vi "getColorMode.vi"(9 "wColorPatternDESC":u16, 10 "wRoiX0":u16, 11 "wRoiY0":u16) -> (3 "colorMode":i32)   [LabVIEW 2020]
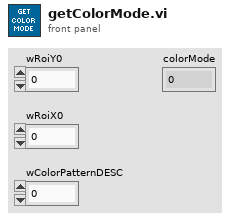
[diagram p1: front panel]
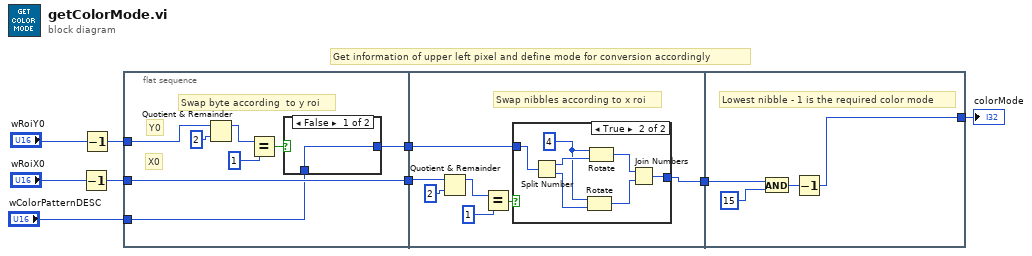
[diagram p0: block diagram]
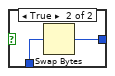
[diagram p2: hidden frame]
diagram:
  # "Get information of upper left pixel and define mode for conversion accordingly"
  n1 = Decrement(x="wRoiX0") -> (x-1=w4:u16)
  n2 = Decrement(x="wRoiY0") -> (x-1=w2:u16)
  n3 = flat-sequence {
    tunnel: w4 -> [w15]
    tunnel: w2 -> [w17]
    tunnel: [w15] -> w9
    tunnel: [w11] -> w8
    tunnel: "wColorPatternDESC" -> [w10]
    tunnel: w9 -> [w24]
    tunnel: w8 -> [w22]
    tunnel: [w21] -> w7
    tunnel: w7 -> [w38]
    tunnel: [w36] -> w1
    frame #0 {
      # "X0"
      # "Y0"
      # "Swap byte according  to y roi"
      n4 = Quotient & Remainder(x=w17, y=u16 2) -> (x-y*floor(x/y)=w14:u16)  [unwired: 1 out]
      n5 = Equal?(x=w14, y=u16 1) -> (x = y?=w12:bool)
      n6 = case shown="False" w12 {
        tunnel: w10 -> [w18 w20]
        tunnel: [w18 w19] -> w11
        frame False {
        }
        frame True {
          n7 = Swap Bytes(anything=w20) -> (byte swapped=w19:u16)
        }
      }
    }
    frame #1 {
      # "Swap nibbles according to x roi"
      n8 = Quotient & Remainder(x=w24, y=u16 2) -> (x-y*floor(x/y)=w26:u16)  [unwired: 1 out]
      n9 = Equal?(x=w26, y=u16 1) -> (x = y?=w23:bool)
      n10 = case shown="True" w23 {
        tunnel: w22 -> [w28 w35]
        tunnel: [w28 w29] -> w21
        frame False {
        }
        frame True {
          w32 = i16 4 ("y")
          n11 = Split Number(x=w35) -> (hi(x)=w33:u8, lo(x)=w34:u8)
          n12 = Rotate(1:w34, 2:w32) -> (0:w30:u8)
          n13 = Rotate(1:w33, 2:w32) -> (0:w31:u8)
          n14 = Join Numbers(hi=w31, lo=w30) -> ((hi.lo)=w29:u16)
        }
      }
    }
    frame #2 {
      # "Lowest nibble - 1 is the required color mode"
      n15 = And(x=w38, y=u16 15) -> (x .and. y?=w37:u16)
      n16 = Decrement(x=w37) -> (x-1=w36:u16)
    }
  }
  "colorMode" <- w1
